vi "Get Scan Mode.vi"(8 "error in (no error)":errorcluster) -> (0 "error out":errorcluster, 2 "mode":i32(ring)=2 items=["Initialization Mode", "Configuration Mode", "Active Mode", "Fault Mode"])   [LabVIEW 2011, in "Scan Engine Custom Device.lvlib"]
uses:
  Scan Engine Custom Device.lvlib
  Program Files (x86)/National Instruments/LabVIEW 2011/resource/objmgr/ni.var.rc
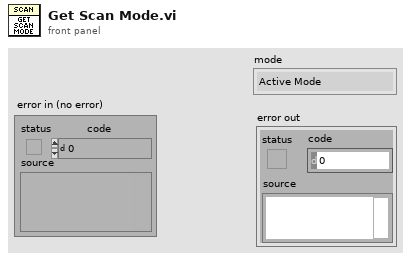
[diagram p1: front panel]
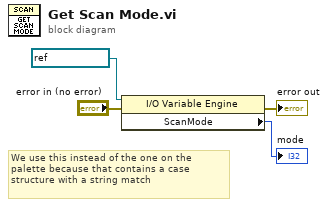
[diagram p0: block diagram]
diagram:
  # "We use this instead of the one on the palette because that contains a case structure with a string match"
  n1 = property class="I/O Variable Engine"(reference=refnum<k21> "ni.var.io:/" ("reference out"), error in="error in (no error)") -> (error out=→"error out":errorcluster, "ScanMode"=→"mode":i32)  [unwired: 1 out]
